vi "Length.vi"(4 "Length":u64, 5 "Mask":bool) -> (7 "Length Data":u8[](array[numeric]) format="%.0x")   [LabVIEW 2020, in "HTTP Server.lvlib" / "WebSocket Client.lvclass"]
uses:
  WebSocket Client.lvclass
  WebSocket Client.lvclass/WebSocket Client.ctl
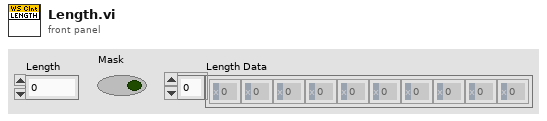
[diagram p1: front panel]
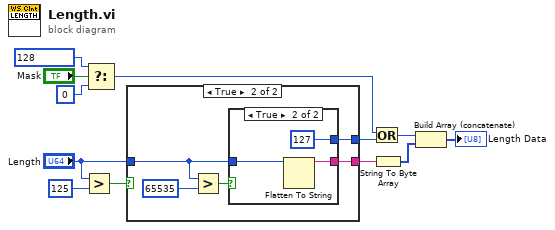
[diagram p0: block diagram]
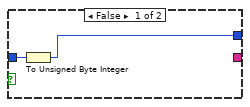
[diagram p2: hidden frame]
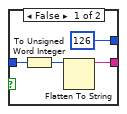
[diagram p3: hidden frame]
diagram:
  n1 = Greater?(x="Length", y=u64 125) -> (0:w11:bool)
  n2 = Select(t=u8 128, s="Mask", f=u8 0) -> (s? t:f=w5:u8)
  n3 = case shown="True" w11 {
    tunnel: "Length" -> [w14 w18]
    tunnel: [_ w16] -> w3
    tunnel: [w13 w15] -> w6
    frame False {
      n4 = To Unsigned Byte Integer(number=w14) -> (unsigned 8bit integer=w13:u8)
    }
    frame True {
      n5 = Greater?(x=w18, y=u64 65535) -> (0:w17:bool)
      n6 = case shown="True" w17 {
        tunnel: w18 -> [w23 w26]
        tunnel: [w21 w25] -> w16
        tunnel: [u8 126 u8 127] -> w15
        frame False {
          n7 = To Unsigned Word Integer(number=w23) -> (unsigned 16bit integer=w22:u16)
          n8 = Flatten To String(anything=w22) -> (data string=w21:string)  [unwired: 3 in, 2 out]
        }
        frame True {
          n9 = Flatten To String(anything=w26) -> (data string=w25:string)  [unwired: 3 in, 2 out]
        }
      }
    }
  }
  n10 = Or(x=w5, y=w6) -> (x .or. y?=w4:u8)
  n11 = String To Byte Array(string=w3) -> (unsigned byte array=w2:u8[])
  n12 = Build Array (concatenate)(w4, w2) -> (→"Length Data":u8[])
